vi "ADIS16470 Loop.vi"(8 "error in":errorcluster) -> ()   [LabVIEW 2025]
uses:
  <vilib>/Rock Robotics/WPI/ThirdParty/ADI/ADIS16470/Typedef/ADIS16470 Device Reference.ctl
  <vilib>/Rock Robotics/WPI/ThirdParty/ADI/ADIS16470/Typedef/ADIS16470 Hardware Configuration.ctl
  <vilib>/Rock Robotics/WPI/SPI/WPI_SPIMode.ctl
  <vilib>/Rock Robotics/SystemInterfaces/DIO/FPGA_DIOChannel.ctl
  <vilib>/Rock Robotics/SystemInterfaces/spilib/spi_bus.ctl
  <vilib>/Rock Robotics/WPI/ThirdParty/ADI/ADIS16470/Typedef/ADIS16470 Status.ctl
  <vilib>/Rock Robotics/WPI/ThirdParty/ADI/ADIS16470/Typedef/ADIS16470 Data.ctl
  <vilib>/Rock Robotics/WPI/ThirdParty/ADI/ADIS16470/Typedef/ADIS16470 Process.ctl
  <vilib>/Rock Robotics/WPI/ThirdParty/ADI/ADIS16470/Typedef/ADIS16470 Command Type.ctl
  <vilib>/Rock Robotics/SystemInterfaces/CounterEncoderSourceConvertion/FPGA_CounterEncoderSourceConvertionLVSourceType.ctl
  <vilib>/Rock Robotics/SystemInterfaces/DIO/FPGA_DIODigitalSourceChannel.ctl
  <vilib>/Rock Robotics/SystemInterfaces/AnalogTrigger/FPGA_AnalogTriggerIndex.ctl
  <vilib>/Rock Robotics/SystemInterfaces/AnalogTrigger/FPGA_AnalogTriggerOutType.ctl
  <vilib>/Rock Robotics/WPI/SPI/WPI_SPIDevRef.ctl
  <vilib>/Rock Robotics/WPI/ThirdParty/ADI/ADIS16470/Typedef/ADIS16470 Register.ctl
  <vilib>/Rock Robotics/WPI/Counter/WPI_CounterDigitalInputToDigitalSource.vi
panel:
  out "Offset Bias":i16[](array[numeric])
  in  "ADIS16470DevRef":T1={"DevStatus"={"status"=FALSE, "code"=0, "source"=""}, "Hardware Config"={"SPI Clock Rate (Hz)"=1000000.0, "IMU SPI Mode (3)"=enum."Mode 3 (Clk Idle High,Sample on Trailing)", "IMU Reset Pin"=enum."SPI Port CS2", "IMU SPI Bus"=enum."SPI On-Board, CS0", "IMU Data Ready Pin"=enum."SPI Port CS1", "Stall Config"={"Pow2BytesPerRead"=255, "StallTicks"=640, "CsToSclkTicks"=5}}, "Calibration Complete"=refnum, "Status Reference"=refnum, "Data Reference"=refnum, "Sychronous Process VI"=refnum, "Cmd FIFO"=refnum, "Source"={"DevStatus"={"status"=FALSE, "code"=0, "source"=""}, "AnalogTriggerMode?"=FALSE, "DigitalMode"={"DIO Channel"=enum."Disabled"}, "AnalogTriggerMode"={"AnalogTriggerIndex"=enum."Trig 0", "OutputType"=enum."InWindow"}}, "Data FIFO"=refnum, "Calibration Time (ms)"=5, "Data Reference"=refnum}
  in  "Main Name":string
  # "XG_BIAS_LOW"
  # "XG_BIAS_HIGH"
  # "YG_BIAS_LOW"
  # "YG_BIAS_HIGH"
  # "ZG_BIAS_LOW"
  # "ZG_BIAS_HIGH"
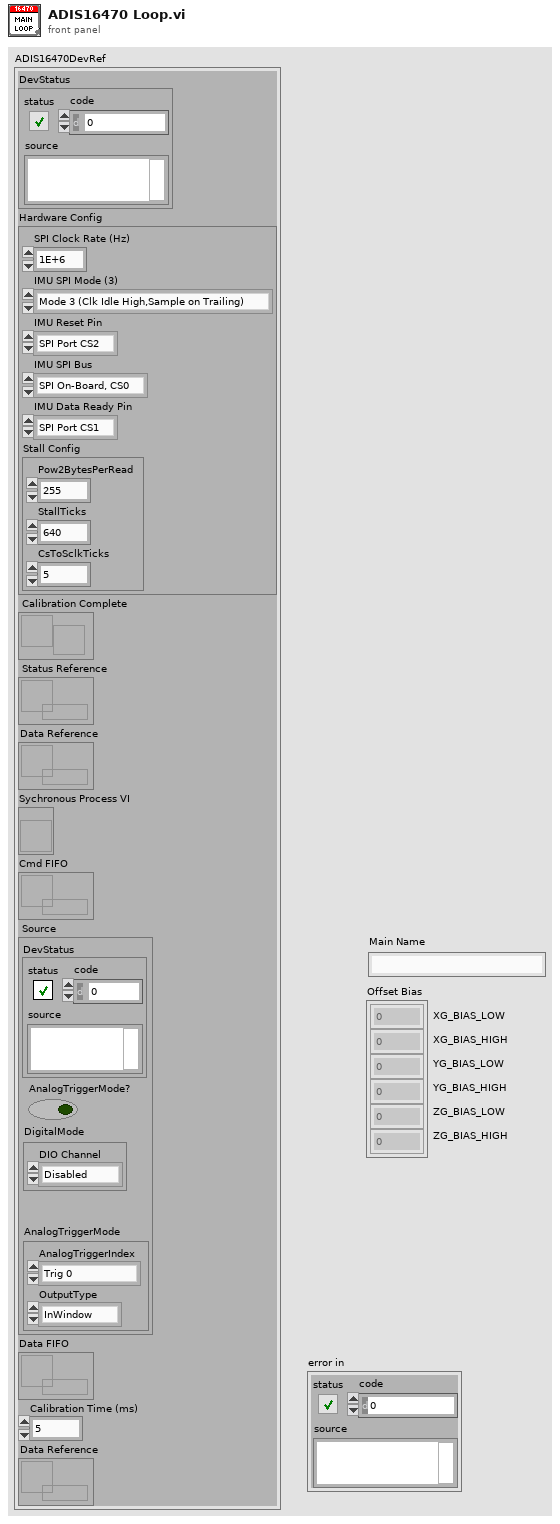
[diagram p1: front panel]
types:
  T1 = typedef "ADIS16470 Device Reference.ctl" = cluster{"DevStatus":errorcluster, "Hardware Config":T2, "Calibration Complete":refnum<notifier>, "Status Reference":refnum<data-value>, "Data Reference":refnum<data-value>, "Sychronous Process VI":T6, "Cmd FIFO":refnum<k33>, "Source":T7, "Data FIFO":refnum<k33>, "Calibration Time (ms)":u32, "Data Reference":refnum<data-value>}
  T2 = typedef "ADIS16470 Hardware Configuration.ctl" = cluster{"SPI Clock Rate (Hz)":dbl, "IMU SPI Mode (3)":T3, "IMU Reset Pin":T4, "IMU SPI Bus":T5, "IMU Data Ready Pin":T4, "Stall Config":cluster{"Pow2BytesPerRead":u8, "StallTicks":u16, "CsToSclkTicks":u8}}
  T3 = typedef "WPI_SPIMode.ctl" = enum16{"Mode 0 (Clk Idle Low,Sample on Leading)", "Mode 1 (Clk Idle Low,Sample on Trailing)", "Mode 2 (Clk Idle High,Sample on Leading)", "Mode 3 (Clk Idle High,Sample on Trailing)"}
  T4 = typedef "FPGA_DIOChannel.ctl" = enum8{"DIO 0", "DIO 1", "DIO 2", "DIO 3", "DIO 4", "DIO 5", "DIO 6", "DIO 7", "DIO 8", "DIO 9", "DIO MXP 0", "DIO MXP 1", "DIO MXP 2", "DIO MXP 3", "DIO MXP 4", "DIO MXP 5", "DIO MXP 6", "DIO MXP 7", "DIO MXP 8", "DIO MXP 9", "DIO MXP 10", "DIO MXP 11", "DIO MXP 12", "DIO MXP 13", "DIO MXP 14", "DIO MXP 15", "SPI Port CS1", "SPI Port CS2", "SPI Port CS3", "SPI Port MISO", "SPI Port MOSI", "Invalid"}
  T5 = typedef "spi_bus.ctl" = enum16{"SPI On-Board, CS0", "SPI On-Board, CS1", "SPI On-Board, CS2", "SPI On-Board, CS3", "SPI MXP", "Invalid"}
  T6 = typedef "ADIS16470 Process.ctl" = refnum<vi>
  T7 = typedef "FPGA_CounterEncoderSourceConvertionLVSourceType.ctl" = cluster{"DevStatus":errorcluster, "AnalogTriggerMode?":bool, "DigitalMode":cluster{"DIO Channel":T8}, "AnalogTriggerMode":cluster{"AnalogTriggerIndex":T9, "OutputType":T10}}
  T8 = typedef "FPGA_DIODigitalSourceChannel.ctl" = enum8{"DIO 0", "DIO 1", "DIO 2", "DIO 3", "DIO 4", "DIO 5", "DIO 6", "DIO 7", "DIO 8", "DIO 9", "DIO MXP 0", "DIO MXP 1", "DIO MXP 2", "DIO MXP 3", "DIO MXP 4", "DIO MXP 5", "DIO MXP 6", "DIO MXP 7", "DIO MXP 8", "DIO MXP 9", "DIO MXP 10", "DIO MXP 11", "DIO MXP 12", "DIO MXP 13", "DIO MXP 14", "DIO MXP 15", "SPI Port CS1", "SPI Port CS2", "SPI Port CS3", "SPI Port MISO", "SPI Port MOSI", "Disabled"}
  T9 = typedef "FPGA_AnalogTriggerIndex.ctl" = enum8{"Trig 0", "Trig 1", "Trig 2", "Trig 3", "Trig 4", "Trig 5", "Trig 6", "Trig 7", "Invalid"}
  T10 = typedef "FPGA_AnalogTriggerOutType.ctl" = enum16{"InWindow", "TriggerState", "Rising", "Falling"}
  T11 = typedef "WPI_SPIDevRef.ctl" = cluster{"DevStatus":errorcluster, "Handle":i32, "SPI Bus":T5}
  T12 = typedef "ADIS16470 Data.ctl" = cluster{"XAngle":dbl, "YAngle":dbl, "ZAngle":dbl}
  T13 = typedef "ADIS16470 Register.ctl" = u8
  T14 = cluster{"SPIDevRef":T11, "Data Counter":u16, "Reset":bool, "Digital Source":T7, "Bytes Per Sample":u32, "Data":T12, "ADIS16470DevRef":T1, "TimeStampPrev":u32, "Sensor to Robot Rotation":dbl[][], "Data Packet":T13[], "AutoSPI Active?":bool, "Delay Factor":dbl}
  T15 = typedef "ADIS16470 Status.ctl" = cluster{"Calibrated?":bool, "IMU Detected?":bool}
  T16 = typedef "ADIS16470 Command Type.ctl" = cluster{"Command":enum16{"None", "Reset", "Recalibrate"}, "Data":u32}
  T17 = typedef "WPI_DigitalOutputDevRef.ctl" = cluster{"DIO Channel":T4, "DevStatus":errorcluster}
  T18 = typedef "WPI_DigitalInputDevRef.ctl" = cluster{"DevStatus":errorcluster, "DIO Channel":T4}
  T19 = cluster{"Pow2BytesPerRead":u8, "StallTicks":u16, "CsToSclkTicks":u8}
  T20 = enum32{"Bad", "Idle", "Run top level", "Running"}
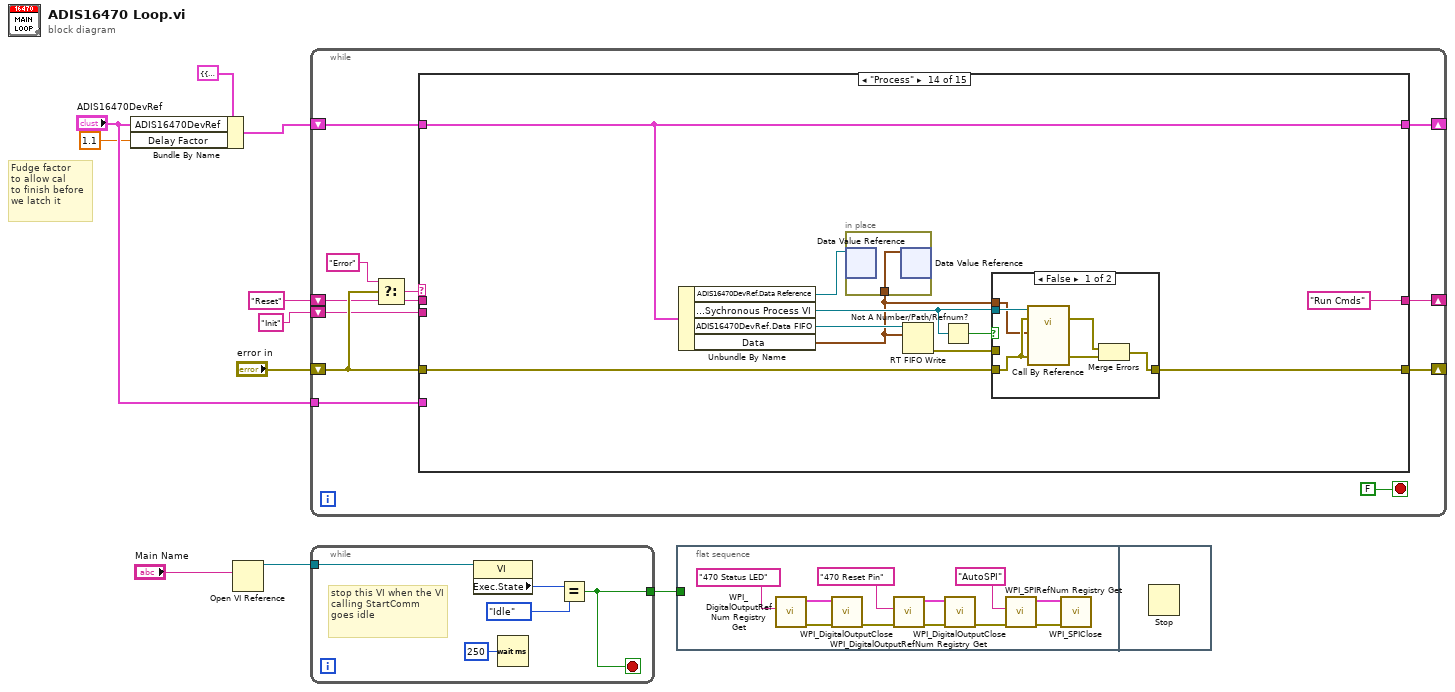
[diagram p0: block diagram]
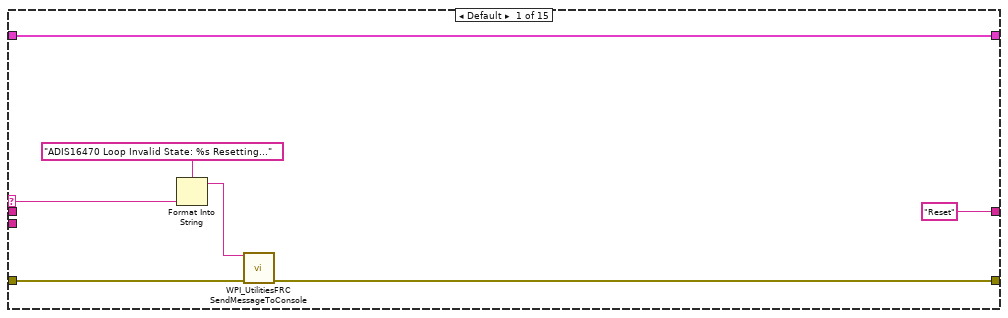
[diagram p2: hidden frame]
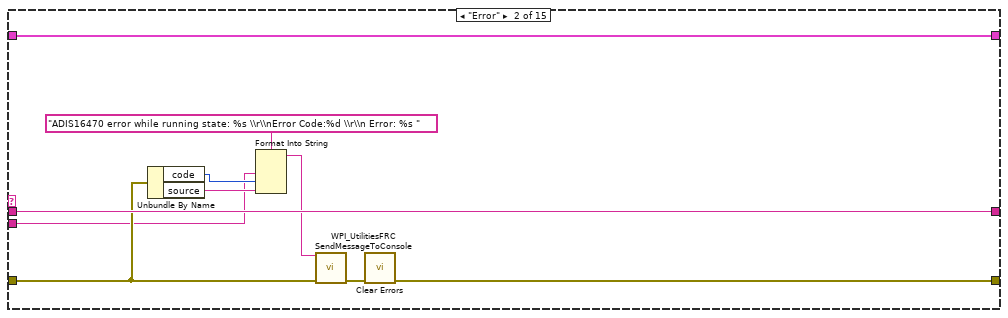
[diagram p3: hidden frame]
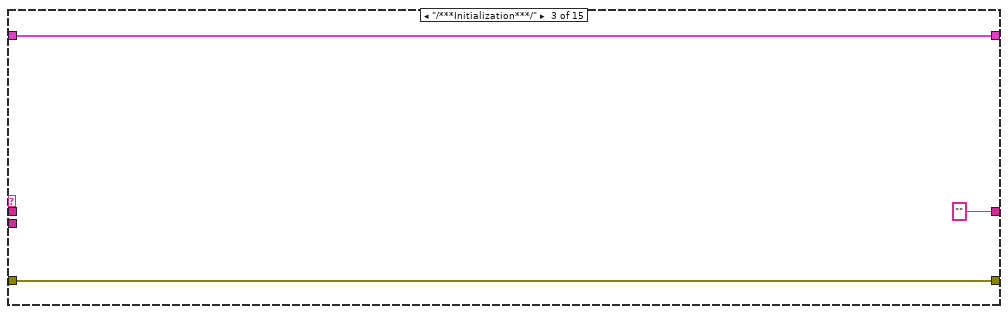
[diagram p4: hidden frame]
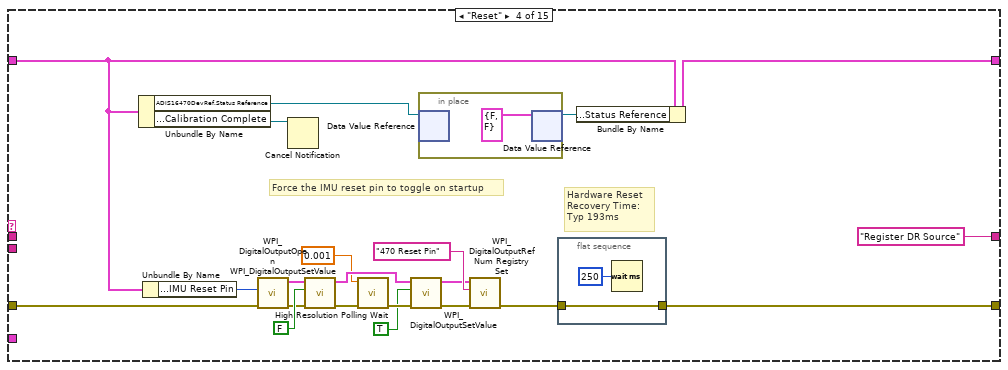
[diagram p5: hidden frame]
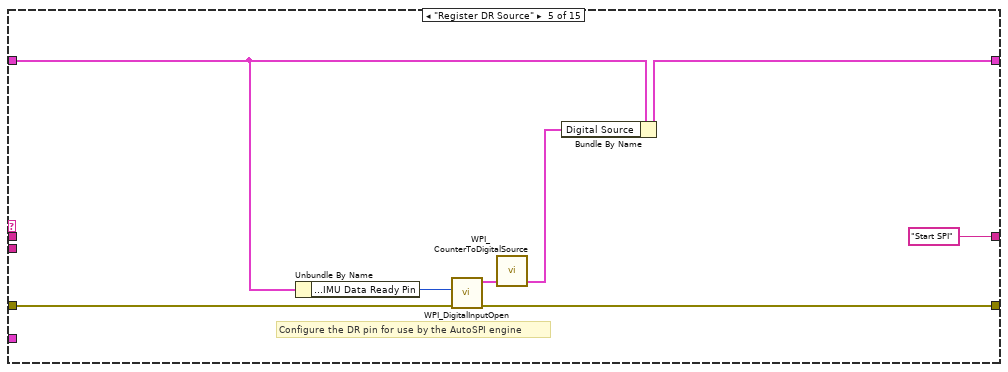
[diagram p6: hidden frame]
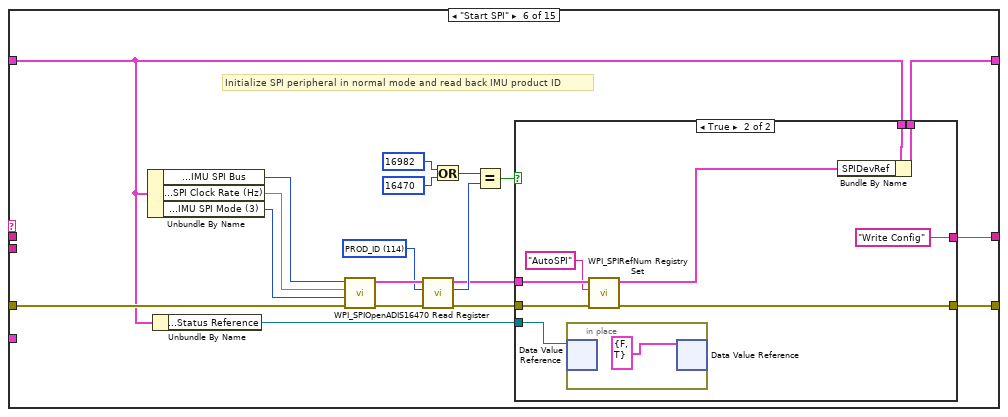
[diagram p7: hidden frame]
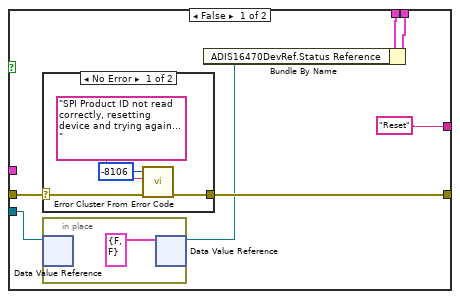
[diagram p8: hidden frame]
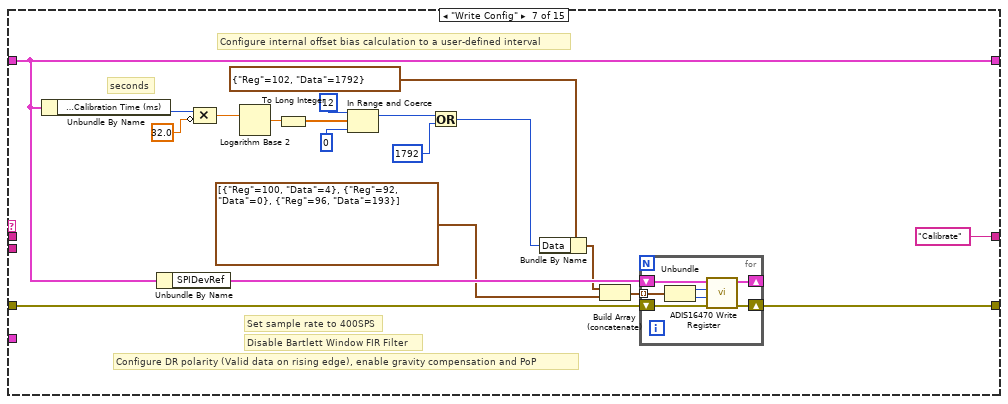
[diagram p10: hidden frame]
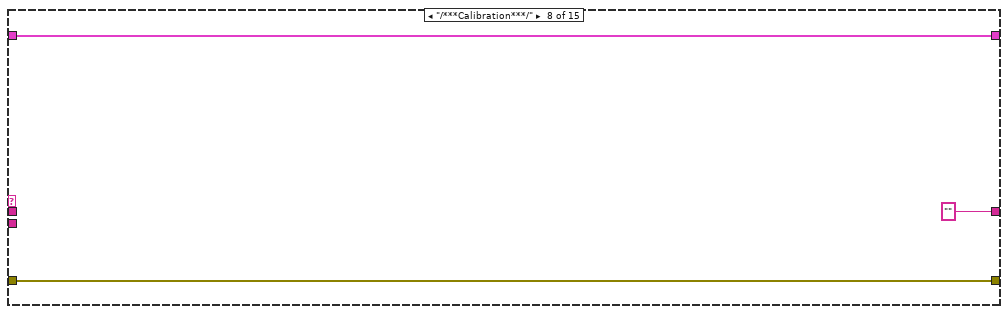
[diagram p11: hidden frame]
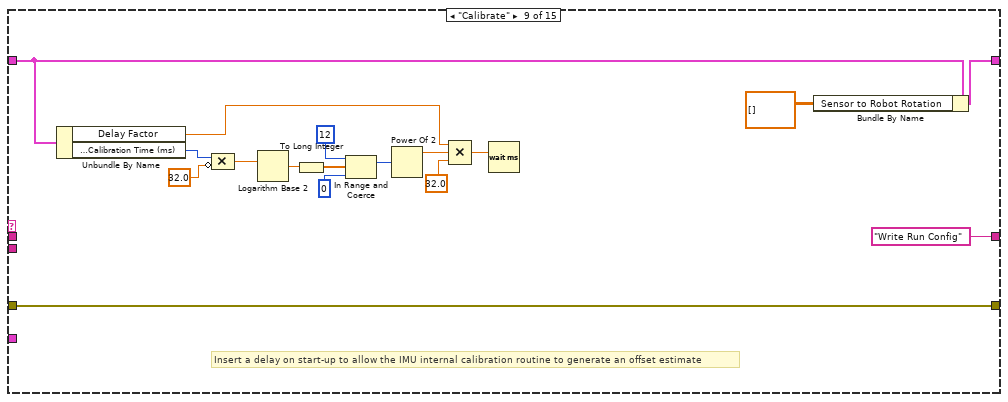
[diagram p12: hidden frame]
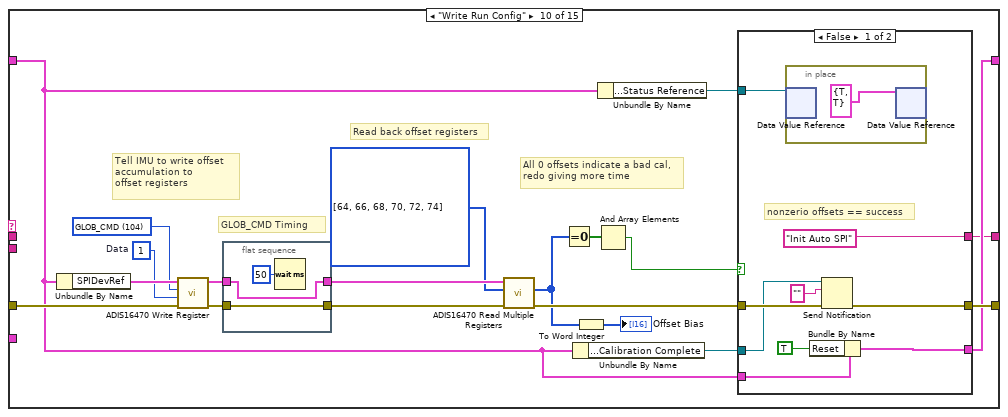
[diagram p13: hidden frame]
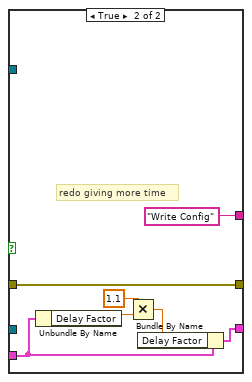
[diagram p14: hidden frame]
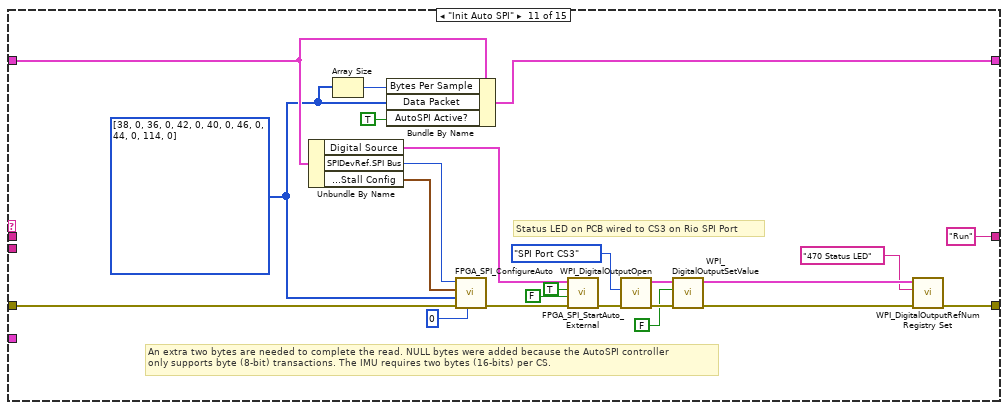
[diagram p15: hidden frame]
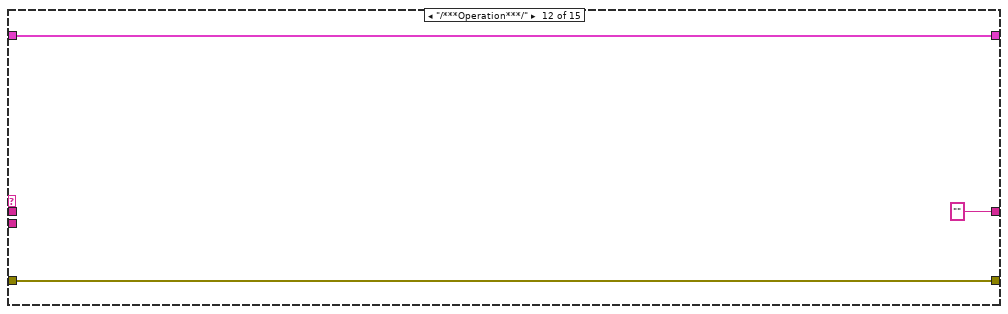
[diagram p16: hidden frame]
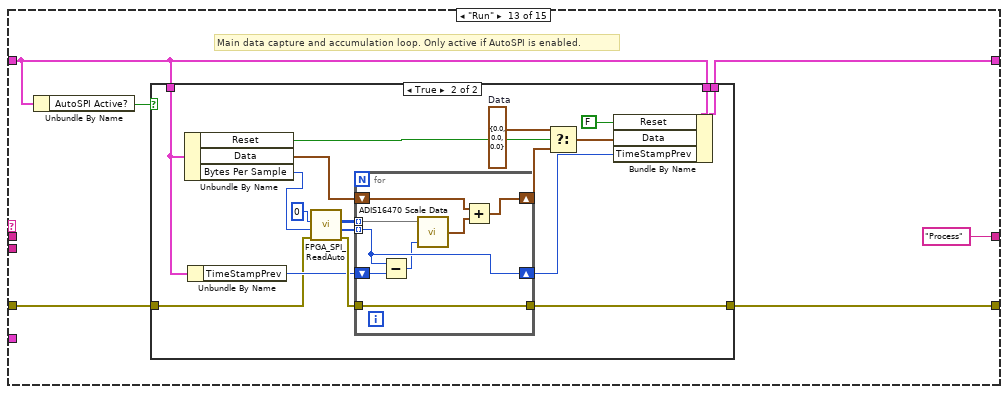
[diagram p17: hidden frame]
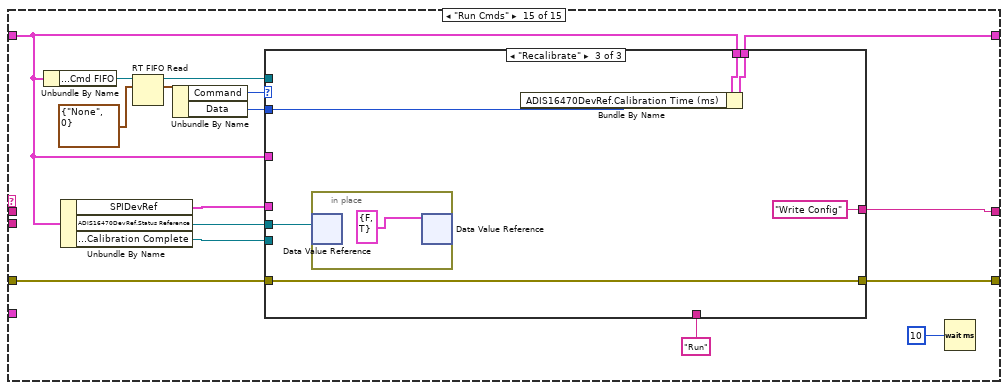
[diagram p20: hidden frame]
diagram:
  # "Fudge factor\nto allow cal\nto finish before\nwe latch it"
  n1 = Bundle By Name(cluster=T14 {"SPIDevRef"={"DevStatus"={"status"=FALSE, "code"=0, "source"=""}, "Handle"=0, "SPI Bus"=enum."SPI On-Board, CS0"}, "Data Counter"=0, "Reset"=FALSE, "Digital Source"={"DevStatus"={"status"=FALSE, "code"=0, "source"=""}, "AnalogTriggerMode?"=FALSE, "DigitalMode"={"DIO Channel"=enum."DIO 1"}, "AnalogTriggerMode"={"AnalogTriggerIndex"=enum."Trig 0", "OutputType"=enum."InWindow"}}, "Bytes Per Sample"=0, "Data"={"XAngle"=0.0, "YAngle"=0.0, "ZAngle"=0.0}, "ADIS16470DevRef"={"DevStatus"={"status"=FALSE, "code"=0, "source"=""}, "Hardware Config"={"SPI Clock Rate (Hz)"=1000000.0, "IMU SPI Mode (3)"=enum."Mode 3 (Clk Idle High,Sample on Trailing)", "IMU Reset Pin"=enum."SPI Port CS2", "IMU SPI Bus"=enum."SPI On-Board, CS0", "IMU Data Ready Pin"=enum."SPI Port CS1", "Stall Config"={"Pow2BytesPerRead"=255, "StallTicks"=640, "CsToSclkTicks"=5}}, "Calibration Complete"=refnum, "Status Reference"=refnum, "Data Reference"=refnum, "Sychronous Process VI"=refnum, "Cmd FIFO"=refnum, "Source"={"DevStatus"={"status"=FALSE, "code"=0, "source"=""}, "AnalogTriggerMode?"=FALSE, "DigitalMode"={"DIO Channel"=enum."Disabled"}, "AnalogTriggerMode"={"AnalogTriggerIndex"=enum."Trig 0", "OutputType"=enum."InWindow"}}, "Data FIFO"=refnum, "Calibration Time (ms)"=5, "Data Reference"=refnum}, "TimeStampPrev"=0, "Sensor to Robot Rotation"=[], "Data Packet"=[38, 0, 36, 0, 42, 0, 40, 0, 46, 0, 44, 0, 114, 0], "AutoSPI Active?"=TRUE, "Delay Factor"=1.1}, "ADIS16470DevRef"="ADIS16470DevRef", "Delay Factor"=1.1) -> (w6:T14)
  n2 = Open VI Reference(vi path="Main Name") -> (vi reference=w9:refnum<vi>)  [unwired: 3 in, 3 out]
  n3 = while {
    shift-right: [w17] -> _
    shift-left: "Reset" -> [w14]
    shift-right: [w19] -> _
    shift-left: w6 -> [w20]
    shift-right: [w18] -> _
    shift-left: "error in" -> [w16]
    shift-left: "Init" -> [w12]
    tunnel: "ADIS16470DevRef" -> [w11]
    stop <- FALSE stop-if-true
    n4 = Select(t="Error", s=w16, f=w14) -> (s? t:f=w15:string)
    n5 = case shown="\"Process\"" w15 {
      selector: w15 -> [w27 _ _ _ _ _ _ _ _ _ _ _ _ _ _]
      tunnel: w20 -> [w28 w38 w41 w45 w69 w75 w124 w144 w157 w164 w216 w227 w229 w270 w284]
      tunnel: [w28 w38 w41 w44 w72 w83 w124 w144 w160 w165 w215 w227 w232 w270 w291] -> w19
      tunnel: w16 -> [w26 w34 w40 w60 w71 w89 w132 w143 w159 w180 w223 w226 w231 w268 w293]
      tunnel: [w25 w35 w40 w58 w66 w82 w131 w143 w159 w171 w207 w226 w230 w267 w292] -> w18
      tunnel: ["Reset" w37 "" "Register DR Source" "Start SPI" w84 "Calibrate" "" "Write Run Config" w163 "Run" "" "Process" "Run Cmds" w281] -> w17
      tunnel: w14 -> [_ w37 _ _ _ _ _ _ _ _ _ _ _ _ _]
      tunnel: w12 -> [_ w29 _ _ _ _ _ _ _ _ _ _ _ _ _]
      tunnel: w11 -> [_ _ _ _ _ _ _ _ _ _ _ _ _ _ _]
      frame Default {
        n6 = Format Into String(format string="ADIS16470 Loop Invalid State: %s Resetting...", w27) -> (resulting string=w24:string)  [unwired: 2 in, 1 out]
        n7 = call <vilib>:"WPI_UtilitiesFRC SendMessageToConsole.vi"("Message"=w24, "error in (no error)"=w26) -> ("error out"=w25:errorcluster)  [unwired: 13 in]
      }
      frame "Error" {
        n8 = Unbundle By Name(w34) -> ("code"=w31:i32, "source"=w30:string)
        n9 = Format Into String(format string="ADIS16470 error while running state: %s \\r\\nError Code:%d \\r\\n Error: %s ", w29, w31, w30) -> (resulting string=w33:string)  [unwired: 2 in, 1 out]
        n10 = call <vilib>:"WPI_UtilitiesFRC SendMessageToConsole.vi"("Message"=w33, "error in (no error)"=w34) -> ("error out"=w36:errorcluster)  [unwired: 13 in]
        n11 = call <vilib>:"Clear Errors.vi"("error in (no error)"=w36) -> ("error out"=w35:errorcluster)  [unwired: 5 in, 1 out]
      }
      frame "/***Initialization***/" {
      }
      frame "Reset" {
        # "Hardware Reset Recovery Time: Typ 193ms"
        # "Force the IMU reset pin to toggle on startup"
        n12 = Unbundle By Name(w45) -> ("ADIS16470DevRef.Status Reference"=w43:refnum<data-value>, "ADIS16470DevRef.Calibration Complete"=w57:refnum<notifier>)
        n13 = Unbundle By Name(w45) -> ("ADIS16470DevRef.Hardware Config.IMU Reset Pin"=w61:T4)
        n14 = call <vilib>:"WPI_DigitalOutputOpen.vi"("error in (no error)"=w60, "DIO Channel"=w61) -> ("error out"=w55:errorcluster, "DigitalOutputDevRef"=w62:T17)  [unwired: 8 in]
        n15 = Cancel Notification(0:w57) -> ()  [unwired: 1 in, 3 out]
        n16 = call <vilib>:"WPI_DigitalOutputSetValue.vi"("error in (no error)"=w55, "Value"=FALSE, "DigitalOutputDevRef"=w62) -> ("error out"=w52:errorcluster, "DigitalOutputDevRef"=w50:T17)  [unwired: 7 in]
        n17 = call <vilib>:"High Resolution Polling Wait.vi"("error in (no error)"=w52, "seconds to wait"=0.001) -> ("error out"=w51:errorcluster)  [unwired: 9 in]
        n18 = call <vilib>:"WPI_DigitalOutputSetValue.vi"("error in (no error)"=w51, "Value"=TRUE, "DigitalOutputDevRef"=w50) -> ("error out"=w47:errorcluster, "DigitalOutputDevRef"=w48:T17)  [unwired: 7 in]
        n19 = in-place {
          n20 = in-place-dvr #1(w43) -> ()  [unwired: 2 out]
          n21 = in-place-dvr #1(T15 {"Calibrated?"=FALSE, "IMU Detected?"=FALSE} ("element")) -> (w42:refnum<data-value>)  [unwired: 1 out]
        }
        n22 = call <vilib>:"WPI_DigitalOutputRefNum Registry Set.vi"("error in (no error)"=w47, "refnum name"="470 Reset Pin", "DigitalOutputDevRef"=w48) -> ("error out"=w53:errorcluster)  [unwired: 7 in, 1 out]
        n23 = flat-sequence {
          tunnel: [w65] -> w58
          tunnel: w53 -> [w65]
          frame #0 {
            n24 = Wait (ms)(milliseconds to wait=u32 250) -> ()  [unwired: 1 out]
          }
        }
        n25 = Bundle By Name(cluster=w45, "ADIS16470DevRef.Status Reference"=w42) -> (w44:T14)
      }
      frame "Register DR Source" {
        # "Configure the DR pin for use by the AutoSPI engine"
        n26 = Unbundle By Name(w69) -> ("ADIS16470DevRef.Hardware Config.IMU Data Ready Pin"=w68:T4)
        n27 = call <vilib>:"WPI_DigitalInputOpen.vi"("error in (no error)"=w71, "DIO Channel"=w68) -> ("error out"=w66:errorcluster, "DigitalInputDevRef"=w70:T18)  [unwired: 8 in]
        n28 = call-poly <vilib>:"WPI_CounterToDigitalSource.vi"("DigitalInputDevRef"=w70) -> ("Digital Source"=w67:T7)  [unwired: 6 in]
        n29 = Bundle By Name(cluster=w69, "Digital Source"=w67) -> (w72:T14)
      }
      frame "Start SPI" {
        w77 = T13 114 items=["Reserved1"=0, "DIAG_STAT"=2, "X_GYRO_LOW"=4, "X_GYRO_OUT"=6, "Y_GYRO_LOW"=8, "Y_GYRO_OUT"=10, "Z_GYRO_LOW"=12, "Z_GYRO_OUT"=14, "X_ACCL_LOW"=16, "X_ACCL_OUT"=18, "Y_ACCL_LOW"=20, "Y_ACCL_OUT"=22, "Z_ACCL_LOW"=24, "Z_ACCL_OUT"=26, "TEMP_OUT"=28, "TIME_STAMP"=30, "Reseved2"=32, "DATA_CNTR"=34, "X_DELTANG_LOW"=36, "X_DELTANG_OUT"=38, "Y_DELTANG_LOW"=40, "Y_DELTANG_OUT"=42, "Z_DELTANG_LOW"=44, "Z_DELTANG_OUT"=46, "X_DELTVEL_LOW"=48, "X_DELTVEL_OUT"=50, "Y_DELTVEL_LOW"=52, "Y_DELTVEL_OUT"=54, "Z_DELTVEL_LOW"=56, "Z_DELTVEL_OUT"=58, "Reserved3"=60, "Reserved4"=62, "XG_BIAS_LOW"=64, "XG_BIAS_HIGH"=66, "YG_BIAS_LOW"=68, "YG_BIAS_OUT"=70, "ZG_BIAS_LOW"=72, "ZG_BIAS_OUT"=74, "XA_BIAS_LOW"=76, "XA_BIAS_HIGH"=78, "YA_BIAS_LOW"=80, "YA_BIAS_OUT"=82, "ZA_BIAS_LOW"=84, "ZA_BIAS_OUT"=86, "Reserved5"=88, "Reserved6"=90, "FILT_CTRL"=92, "Reserved5"=94, "MSC_CTRL"=96, "UP_SCALE"=98, "DEC_RATE"=100, "NULL_CNFG"=102, "GLOB_CMD"=104, "Reserved6"=106, "FIRM_REV"=108, "FIRM_DM"=110, "FIRM_Y"=112, "PROD_ID"=114, "SERIAL_NUM"=116, "USER_SCR1"=118, "USER_SCR2"=120, "USER_SCR3"=122, "FLSHCNT_LOW"=124, "FLSHCNT_HIGH"=126] ("ADIS16448 Register")
        # "Initialize SPI peripheral in normal mode and read back IMU product ID"
        n30 = Unbundle By Name(w75) -> ("ADIS16470DevRef.Hardware Config.IMU SPI Bus"=w85:T5, "ADIS16470DevRef.Hardware Config.SPI Clock Rate (Hz)"=w86:dbl, "ADIS16470DevRef.Hardware Config.IMU SPI Mode (3)"=w87:T3)
        n31 = Unbundle By Name(w75) -> ("ADIS16470DevRef.Status Reference"=w74:refnum<data-value>)
        n32 = call <vilib>:"WPI_SPIOpen.vi"("error in"=w89, "Mode (3)"=w87, "Clock Rate (Hz)"=w86, "SPI Bus"=w85) -> ("error out"=w79:errorcluster, "SPIDevRef"=w78:T11)  [unwired: 6 in]
        n33 = call <vilib>:"ADIS16470 Read Register.vi"("error in (no error)"=w79, "ADIS16470 Register"=w77, "SPIDevRef in"=w78) -> ("error out"=w80:errorcluster, "Register Value"=w81:u16, "SPIDevRef out"=w76:T11)  [unwired: 6 in]
        n34 = Or(x=u16 16982 ("y"), y=u16 16470) -> (x .or. y?=w90:u16)
        n35 = Equal?(x=w90, y=w81) -> (x = y?=w88:bool)
        n36 = case shown="True" w88 {
          tunnel: ["Reset" "Write Config"] -> w84
          tunnel: w75 -> [w95 w113]
          tunnel: [w94 w112] -> w83
          tunnel: [w98 w108] -> w82
          tunnel: w80 -> [w97 w111]
          tunnel: w76 -> [_ w110]
          tunnel: w74 -> [w96 w106]
          frame False {
            n37 = case shown="No Error" w97 {
              selector: w97 -> [w103 w105]
              tunnel: [w104 w105] -> w98
              frame No Error {
                n38 = call <vilib>:"Error Cluster From Error Code.vi"("error in (no error)"=w103, "error message (\"\")"="SPI Product ID not read correctly, resetting device and trying again..." ("error message (\"\")"), "error code (0)"=-8106) -> ("error out"=w104:errorcluster)  [unwired: 6 in]
              }
              frame Error {
              }
            }
            n39 = in-place {
              n40 = in-place-dvr #2(w96) -> ()  [unwired: 2 out]
              n41 = in-place-dvr #2(T15 {"Calibrated?"=FALSE, "IMU Detected?"=FALSE} ("element")) -> (w93:refnum<data-value>)  [unwired: 1 out]
            }
            n42 = Bundle By Name(cluster=w95, "ADIS16470DevRef.Status Reference"=w93) -> (w94:T14)
          }
          frame True {
            n43 = in-place {
              n44 = in-place-dvr #3(w106) -> ()  [unwired: 2 out]
              n45 = in-place-dvr #3(T15 {"Calibrated?"=FALSE, "IMU Detected?"=TRUE} ("element")) -> ()  [unwired: 2 out]
            }
            n46 = call <vilib>:"WPI_SPIRefNum Registry Set.vi"("error in (no error)"=w111, "refnum name"="AutoSPI", "SPIDevRef"=w110) -> ("error out"=w108:errorcluster, "SPIDevRef"=w109:T11)  [unwired: 7 in]
            n47 = Bundle By Name(cluster=w113, "SPIDevRef"=w109) -> (w112:T14)
          }
        }
      }
      frame "Write Config" {
        # "seconds"
        # "Set sample rate to 400SPS"
        # "Configure internal offset bias calculation to a user-defined interval"
        # "Configure DR polarity (Valid data on rising edge), enable gravity compensation and PoP"
        # "Disable Bartlett Window FIR Filter"
        n48 = Unbundle By Name(w124) -> ("ADIS16470DevRef.Calibration Time (ms)"=w119:u32)
        n49 = Unbundle By Name(w124) -> ("SPIDevRef"=w133:T11)
        n50 = Compound Arithmetic op=MULTIPLY(w119, invert 32.0 ("x")) -> (w117:dbl)
        n51 = Logarithm Base 2(1:w117) -> (0:w123:dbl)
        n52 = To Long Integer(number=w123) -> (32bit integer=w120:i32)
        n53 = In Range and Coerce(upper limit=12 ("x"), x=w120, lower limit=0 ("x")) -> (coerced(x)=w116:i32)  [unwired: 1 out]
        n54 = Or(x=w116, y=1792 ("Data")) -> (x .or. y?=w125:i32)
        n55 = Bundle By Name(cluster=cluster{"Reg":T13, "Data":i32} {"Reg"=102, "Data"=1792}, "Data"=w125) -> (w127:cluster{"Reg":T13, "Data":i32})
        n56 = Build Array (concatenate)(w127, cluster{"Reg":T13, "Data":u16}[] [{"Reg"=100, "Data"=4}, {"Reg"=92, "Data"=0}, {"Reg"=96, "Data"=193}]) -> (w128:cluster{"Reg":T13, "Data":i32}[])
        n57 = for {
          tunnel: w128 -> [w141] mode=indexing
          shift-right: [w137] -> w131
          shift-left: w132 -> [w136]
          shift-right: [w135] -> _
          shift-left: w133 -> [w138]
          n58 = Unbundle(w141) -> ("Reg"=w140:T13, "Data"=w139:i32)
          n59 = call <vilib>:"ADIS16470 Write Register.vi"("error in (no error)"=w136, "Data"=w139, "Register"=w140, "SPIDevRef in"=w138) -> ("error out"=w137:errorcluster, "SPIDevRef out"=w135:T11)  [unwired: 6 in]
        }
      }
      frame "/***Calibration***/" {
      }
      frame "Calibrate" {
        # "Insert a delay on start-up to allow the IMU internal calibration routine to generate an offset estimate"
        n60 = Unbundle By Name(w157) -> ("Delay Factor"=w145:dbl, "ADIS16470DevRef.Calibration Time (ms)"=w151:u32)
        n61 = Compound Arithmetic op=MULTIPLY(w151, invert 32.0 ("x")) -> (w152:dbl)
        n62 = Logarithm Base 2(1:w152) -> (0:w156:dbl)
        n63 = To Long Integer(number=w156) -> (32bit integer=w154:i32)
        n64 = In Range and Coerce(upper limit=12 ("x"), x=w154, lower limit=0 ("x")) -> (coerced(x)=w149:i32)  [unwired: 1 out]
        n65 = Power Of 2(x=w149) -> (2^x=w148:dbl)
        n66 = Compound Arithmetic op=MULTIPLY(w145, w148, 32.0 ("x")) -> (w146:dbl)
        n67 = Wait (ms)(milliseconds to wait=w146) -> ()  [unwired: 1 out]
        n68 = Bundle By Name(cluster=w157, "Sensor to Robot Rotation"=dbl[][] []) -> (w160:T14)
      }
      frame "Write Run Config" {
        w170 = T13 104 items=["Reserved1"=0, "DIAG_STAT"=2, "X_GYRO_LOW"=4, "X_GYRO_OUT"=6, "Y_GYRO_LOW"=8, "Y_GYRO_OUT"=10, "Z_GYRO_LOW"=12, "Z_GYRO_OUT"=14, "X_ACCL_LOW"=16, "X_ACCL_OUT"=18, "Y_ACCL_LOW"=20, "Y_ACCL_OUT"=22, "Z_ACCL_LOW"=24, "Z_ACCL_OUT"=26, "TEMP_OUT"=28, "TIME_STAMP"=30, "Reseved2"=32, "DATA_CNTR"=34, "X_DELTANG_LOW"=36, "X_DELTANG_OUT"=38, "Y_DELTANG_LOW"=40, "Y_DELTANG_OUT"=42, "Z_DELTANG_LOW"=44, "Z_DELTANG_OUT"=46, "X_DELTVEL_LOW"=48, "X_DELTVEL_OUT"=50, "Y_DELTVEL_LOW"=52, "Y_DELTVEL_OUT"=54, "Z_DELTVEL_LOW"=56, "Z_DELTVEL_OUT"=58, "Reserved3"=60, "Reserved4"=62, "XG_BIAS_LOW"=64, "XG_BIAS_HIGH"=66, "YG_BIAS_LOW"=68, "YG_BIAS_OUT"=70, "ZG_BIAS_LOW"=72, "ZG_BIAS_OUT"=74, "XA_BIAS_LOW"=76, "XA_BIAS_HIGH"=78, "YA_BIAS_LOW"=80, "YA_BIAS_OUT"=82, "ZA_BIAS_LOW"=84, "ZA_BIAS_OUT"=86, "Reserved5"=88, "Reserved6"=90, "FILT_CTRL"=92, "Reserved5"=94, "MSC_CTRL"=96, "UP_SCALE"=98, "DEC_RATE"=100, "NULL_CNFG"=102, "GLOB_CMD"=104, "Reserved6"=106, "FIRM_REV"=108, "FIRM_DM"=110, "FIRM_Y"=112, "PROD_ID"=114, "SERIAL_NUM"=116, "USER_SCR1"=118, "USER_SCR2"=120, "USER_SCR3"=122, "FLSHCNT_LOW"=124, "FLSHCNT_HIGH"=126] ("Register")
        w179 = u16 1  # Data
        w175 = T13[] [64, 66, 68, 70, 72, 74] items=["Reserved1"=0, "DIAG_STAT"=2, "X_GYRO_LOW"=4, "X_GYRO_OUT"=6, "Y_GYRO_LOW"=8, "Y_GYRO_OUT"=10, "Z_GYRO_LOW"=12, "Z_GYRO_OUT"=14, "X_ACCL_LOW"=16, "X_ACCL_OUT"=18, "Y_ACCL_LOW"=20, "Y_ACCL_OUT"=22, "Z_ACCL_LOW"=24, "Z_ACCL_OUT"=26, "TEMP_OUT"=28, "TIME_STAMP"=30, "Reseved2"=32, "DATA_CNTR"=34, "X_DELTANG_LOW"=36, "X_DELTANG_OUT"=38, "Y_DELTANG_LOW"=40, "Y_DELTANG_OUT"=42, "Z_DELTANG_LOW"=44, "Z_DELTANG_OUT"=46, "X_DELTVEL_LOW"=48, "X_DELTVEL_OUT"=50, "Y_DELTVEL_LOW"=52, "Y_DELTVEL_OUT"=54, "Z_DELTVEL_LOW"=56, "Z_DELTVEL_OUT"=58, "Reserved3"=60, "Reserved4"=62, "XG_BIAS_LOW"=64, "XG_BIAS_HIGH"=66, "YG_BIAS_LOW"=68, "YG_BIAS_HIGH"=70, "ZG_BIAS_LOW"=72, "ZG_BIAS_HIGH"=74, "XA_BIAS_LOW"=76, "XA_BIAS_HIGH"=78, "YA_BIAS_LOW"=80, "YA_BIAS_HIGH"=82, "ZA_BIAS_LOW"=84, "ZA_BIAS_HIGH"=86, "Reserved5"=88, "Reserved6"=90, "FILT_CTRL"=92, "Reserved5"=94, "MSC_CTRL"=96, "UP_SCALE"=98, "DEC_RATE"=100, "NULL_CNFG"=102, "GLOB_CMD"=104, "Reserved6"=106, "FIRM_REV"=108, "FIRM_DM"=110, "FIRM_Y"=112, "PROD_ID"=114, "SERIAL_NUM"=116, "USER_SCR1"=118, "USER_SCR2"=120, "USER_SCR3"=122, "FLSHCNT_LOW"=124, "FLSHCNT_HIGH"=126] ("Registers")
        # "All 0 offsets indicate a bad cal,\nredo giving more time"
        # "Tell IMU to write offset \naccumulation to \noffset registers"
        # "GLOB_CMD Timing"
        # "Read back offset registers"
        n69 = Unbundle By Name(w164) -> ("SPIDevRef"=w181:T11)
        n70 = call <vilib>:"ADIS16470 Write Register.vi"("error in (no error)"=w180, "Data"=w179, "Register"=w170, "SPIDevRef in"=w181) -> ("error out"=w178:errorcluster, "SPIDevRef out"=w177:T11)  [unwired: 6 in]
        n71 = flat-sequence {
          tunnel: w178 -> [w201]
          tunnel: [w201] -> w169
          tunnel: w177 -> [w199]
          tunnel: [w199] -> w176
          frame #0 {
            n72 = Wait (ms)(milliseconds to wait=u32 50) -> ()  [unwired: 1 out]
          }
        }
        n73 = call <vilib>:"ADIS16470 Read Multiple Registers.vi"("error in (no error)"=w169, "Registers"=w175, "SPIDevRefIn"=w176) -> ("error out"=w173:errorcluster, "Values"=w168:u16[])  [unwired: 6 in, 1 out]
        n74 = Equal To 0?(x=w168) -> (x = 0?=w167:bool[])
        n75 = Unbundle By Name(w164) -> ("ADIS16470DevRef.Calibration Complete"=w172:refnum<notifier>)
        n76 = To Word Integer(number=w168) -> (16bit integer=→"Offset Bias":i16[])
        n77 = Unbundle By Name(w164) -> ("ADIS16470DevRef.Status Reference"=w162:refnum<data-value>)
        n78 = And Array Elements(Boolean array=w167) -> (logical AND=w166:bool)
        n79 = case shown="False" w166 {
          tunnel: w173 -> [w190 w198]
          tunnel: w172 -> [w189 _]
          tunnel: [w188 w198] -> w171
          tunnel: w164 -> [w185 w196]
          tunnel: [w184 w197] -> w165
          tunnel: ["Init Auto SPI" "Write Config"] -> w163
          tunnel: w162 -> [w182 _]
          frame False {
            # "nonzerio offsets == success"
            n80 = in-place {
              n81 = in-place-dvr #4(w182) -> ()  [unwired: 2 out]
              n82 = in-place-dvr #4(T15 {"Calibrated?"=TRUE, "IMU Detected?"=TRUE} ("element")) -> ()  [unwired: 2 out]
            }
            n83 = Bundle By Name(cluster=w185, "Reset"=TRUE ("First Run")) -> (w184:T14)
            n84 = Send Notification(notification="", notifier=w189, error in (no error)=w190) -> (error out=w188:errorcluster)  [unwired: 1 out]
          }
          frame True {
            # "redo giving more time"
            n85 = Unbundle By Name(w196) -> ("Delay Factor"=w195:dbl)
            n86 = Multiply(x=1.1, y=w195) -> (x*y=w193:dbl)
            n87 = Bundle By Name(cluster=w196, "Delay Factor"=w193) -> (w197:T14)
          }
        }
      }
      frame "Init Auto SPI" {
        w202 = T13[] [38, 0, 36, 0, 42, 0, 40, 0, 46, 0, 44, 0, 114, 0] items=["NULL"=0, "DIAG_STAT"=2, "X_GYRO_LOW"=4, "X_GYRO_OUT"=6, "Y_GYRO_LOW"=8, "Y_GYRO_OUT"=10, "Z_GYRO_LOW"=12, "Z_GYRO_OUT"=14, "X_ACCL_LOW"=16, "X_ACCL_OUT"=18, "Y_ACCL_LOW"=20, "Y_ACCL_OUT"=22, "Z_ACCL_LOW"=24, "Z_ACCL_OUT"=26, "TEMP_OUT"=28, "TIME_STAMP"=30, "Reseved2"=32, "DATA_CNTR"=34, "X_DELTANG_LOW"=36, "X_DELTANG_OUT"=38, "Y_DELTANG_LOW"=40, "Y_DELTANG_OUT"=42, "Z_DELTANG_LOW"=44, "Z_DELTANG_OUT"=46, "X_DELTVEL_LOW"=48, "X_DELTVEL_OUT"=50, "Y_DELTVEL_LOW"=52, "Y_DELTVEL_OUT"=54, "Z_DELTVEL_LOW"=56, "Z_DELTVEL_OUT"=58, "Reserved3"=60, "Reserved4"=62, "XG_BIAS_LOW"=64, "XG_BIAS_HIGH"=66, "YG_BIAS_LOW"=68, "YG_BIAS_HIGH"=70, "ZG_BIAS_LOW"=72, "ZG_BIAS_HIGH"=74, "XA_BIAS_LOW"=76, "XA_BIAS_HIGH"=78, "YA_BIAS_LOW"=80, "YA_BIAS_HIGH"=82, "ZA_BIAS_LOW"=84, "ZA_BIAS_HIGH"=86, "Reserved5"=88, "Reserved6"=90, "FILT_CTRL"=92, "Reserved5"=94, "MSC_CTRL"=96, "UP_SCALE"=98, "DEC_RATE"=100, "NULL_CNFG"=102, "GLOB_CMD"=104, "Reserved6"=106, "FIRM_REV"=108, "FIRM_DM"=110, "FIRM_Y"=112, "PROD_ID"=114, "SERIAL_NUM"=116, "USER_SCR1"=118, "USER_SCR2"=120, "USER_SCR3"=122, "FLSHCNT_LOW"=124, "FLSHCNT_HIGH"=126] ("Registers")
        # "Status LED on PCB wired to CS3 on Rio SPI Port"
        # "An extra two bytes are needed to complete the read. NULL bytes were added because the AutoSPI controller \nonly supports byte (8-bit) transactions. The IMU requires two bytes (16-bits) per CS."
        n88 = Unbundle By Name(w216) -> ("Digital Source"=w204:T7, "SPIDevRef.SPI Bus"=w203:T5, "ADIS16470DevRef.Hardware Config.Stall Config"=w206:T19)
        n89 = Array Size(array=w202) -> (size(s)=w214:i32)
        n90 = Bundle By Name(cluster=w216, "Bytes Per Sample"=w214, "Data Packet"=w202, "AutoSPI Active?"=TRUE) -> (w215:T14)
        n91 = call <vilib>:"FPGA_SPI_ConfigureAuto.vi"("SPI Auto Zero Byte Count"=u8 0, "error in"=w223, "SPI Auto TX Byte Array"=w202, "Stall Config"=w206, "SPI Bus"=w203) -> ("error out"=w221:errorcluster)  [unwired: 6 in]
        n92 = call <vilib>:"FPGA_SPI_StartAuto_External.vi"("error in (no error)"=w221, "Falling Edge"=FALSE, "Rising Edge"=TRUE, "Source"=w204) -> ("error out"=w217:errorcluster)  [unwired: 7 in]
        n93 = call <vilib>:"WPI_DigitalOutputOpen.vi"("error in (no error)"=w217, "DIO Channel"=FPGA_DIOChannel."SPI Port CS3") -> ("error out"=w213:errorcluster, "DigitalOutputDevRef"=w212:T17)  [unwired: 8 in]
        n94 = call <vilib>:"WPI_DigitalOutputSetValue.vi"("error in (no error)"=w213, "Value"=FALSE, "DigitalOutputDevRef"=w212) -> ("error out"=w210:errorcluster, "DigitalOutputDevRef"=w209:T17)  [unwired: 7 in]
        n95 = call <vilib>:"WPI_DigitalOutputRefNum Registry Set.vi"("error in (no error)"=w210, "refnum name"="470 Status LED", "DigitalOutputDevRef"=w209) -> ("error out"=w207:errorcluster)  [unwired: 7 in, 1 out]
      }
      frame "/***Operation***/" {
      }
      frame "Run" {
        # "Main data capture and accumulation loop. Only active if AutoSPI is enabled."
        n96 = Unbundle By Name(w229) -> ("AutoSPI Active?"=w228:bool)
        n97 = case shown="True" w228 {
          tunnel: [w235 w253] -> w232
          tunnel: w231 -> [w234 w238]
          tunnel: [w234 w243] -> w230
          tunnel: w229 -> [w235 w242]
          tunnel: w229 -> [_ w239]
          frame False {
          }
          frame True {
            w237 = T12 {"XAngle"=0.0, "YAngle"=0.0, "ZAngle"=0.0}  # Data
            n98 = Unbundle By Name(w239) -> ("Reset"=w251:bool, "Data"=w246:T12, "Bytes Per Sample"=w250:u32)
            n99 = Unbundle By Name(w239) -> ("TimeStampPrev"=w241:u32)
            n100 = call <vilib>:"FPGA_SPI_ReadAuto.vi"("error in (no error)"=w238, "Bytes per Sample"=w250, "Samples to Read"=u32 0) -> ("error out"=w244:errorcluster, "Timestamps"=w247:u32[], "Data"=w248:u8[][])  [unwired: 6 in]
            n101 = for {
              tunnel: w248 -> [w257] mode=indexing
              tunnel: w247 -> [w259] mode=indexing
              shift-right: [w256] -> w245
              shift-left: w246 -> [w261]
              tunnel: w244 -> [w258]
              tunnel: [w258] -> w243
              shift-right: [w259] -> w240
              shift-left: w241 -> [w260]
              n102 = Subtract(x=w259, y=w260) -> (x-y=w254:u32)
              n103 = call <vilib>:"ADIS16470 Scale Data.vi"("TimeStamp"=w254, "Data In"=w257) -> ("Data"=w255:T12)  [unwired: 3 in]
              n104 = Add(x=w261, y=w255) -> (x+y=w256:T12)
            }
            n105 = Select(t=w237, s=w251, f=w245) -> (s? t:f=w236:T12)
            n106 = Bundle By Name(cluster=w242, "Reset"=FALSE ("First Run"), "Data"=w236, "TimeStampPrev"=w240) -> (w253:T14)
          }
        }
      }
      frame "Process" {
        n107 = Unbundle By Name(w270) -> ("ADIS16470DevRef.Data Reference"=w264:refnum<data-value>, "ADIS16470DevRef.Sychronous Process VI"=w265:T6, "ADIS16470DevRef.Data FIFO"=w269:refnum<k33>, "Data"=w262:T12)
        n108 = in-place {
          in-place-border: w262 -> [w272]
          n109 = in-place-dvr #5(w264) -> ()  [unwired: 2 out]
          n110 = in-place-dvr #5(w272) -> ()  [unwired: 2 out]
        }
        n111 = RT FIFO Write(0:w269, 1:w262) -> (11:w263:errorcluster)  [unwired: 3 in, 3 out]
        n112 = Not A Number/Path/Refnum?(number/path/refnum=w265) -> (NaN/Path/Refnum?=w266:bool)
        n113 = case shown="False" w266 {
          tunnel: w268 -> [w274 w279]
          tunnel: [w278 w279] -> w267
          tunnel: w265 -> [w277 _]
          tunnel: w263 -> [_ _]
          tunnel: w262 -> [w273 _]
          frame False {
            n114 = call-by-ref "?"(reference=w277, error in=w274, 8:"error in (no error)"=w274, "element"=w273) -> (error out=w275:errorcluster, 0:"error out"=w276:errorcluster)  [unwired: 9 in, 1 out]
            n115 = Merge Errors(w275, w276) -> (w278:errorcluster)
          }
          frame True {
          }
        }
      }
      frame "Run Cmds" {
        n116 = Unbundle By Name(w284) -> ("ADIS16470DevRef.Cmd FIFO"=w294:refnum<k33>)
        n117 = Unbundle By Name(w284) -> ("SPIDevRef"=w283:T11, "ADIS16470DevRef.Status Reference"=w289:refnum<data-value>, "ADIS16470DevRef.Calibration Complete"=w290:refnum<notifier>)
        n118 = RT FIFO Read(0:w294, 1:T16 {"Command"=enum."None", "Data"=0} ("element")) -> (8:w288:refnum<k33>, 9:w287:T16)  [unwired: 2 in, 3 out]
        n119 = Unbundle By Name(w287) -> ("Command"=w286:enum16{"None", "Reset", "Recalibrate"}, "Data"=w285:u32)
        n120 = case shown="\"Recalibrate\"" w286 {
          tunnel: w284 -> [w297 w303 w306]
          tunnel: w293 -> [w298 w302 w308]
          tunnel: [w298 w302 w308] -> w292
          tunnel: [w297 w301 w307] -> w291
          tunnel: w290 -> [_ _ _]
          tunnel: w289 -> [_ _ w304]
          tunnel: w288 -> [_ _ _]
          tunnel: w285 -> [_ _ w305]
          tunnel: w284 -> [_ _ _]
          tunnel: w283 -> [_ _ _]
          tunnel: [w296 "Run" "Write Config"] -> w281
          tunnel: "Run" -> [w296 _ _]
          frame "None", Default {
          }
          frame "Reset" {
            n121 = Bundle By Name(cluster=w303, "Reset"=TRUE ("First Run")) -> (w301:T14)
          }
          frame "Recalibrate" {
            n122 = in-place {
              n123 = in-place-dvr #6(w304) -> ()  [unwired: 2 out]
              n124 = in-place-dvr #6(T15 {"Calibrated?"=FALSE, "IMU Detected?"=TRUE} ("element")) -> ()  [unwired: 2 out]
            }
            n125 = Bundle By Name(cluster=w306, "ADIS16470DevRef.Calibration Time (ms)"=w305) -> (w307:T14)
          }
        }
        n126 = Wait (ms)(milliseconds to wait=u32 10) -> ()  [unwired: 1 out]
      }
    }
  }
  n127 = while {
    tunnel: w9 -> [w312]
    tunnel: [w311] -> w3
    stop <- w311 stop-if-true
    # "stop this VI when the VI calling StartComm goes idle"
    n128 = property class="VI"(reference=w312) -> ("Exec.State"=w314:T20)  [unwired: 1 in, 2 out]
    n129 = Wait (ms)(milliseconds to wait=u32 250) -> ()  [unwired: 1 out]
    n130 = Equal?(x=w314, y=T20."Idle" ("Execution:State")) -> (x = y?=w311:bool)
  }
  n131 = flat-sequence {
    tunnel: w3 -> [_]
    frame #0 {
      n132 = call <vilib>:"WPI_DigitalOutputRefNum Registry Get.vi"("refnum name"="470 Status LED") -> ("error out"=w325:errorcluster, "DigitalOutputDevRef"=w324:T17)  [unwired: 9 in]
      n133 = call <vilib>:"WPI_DigitalOutputClose.vi"("error in (no error)"=w325, "DigitalOutputDevRef"=w324) -> ("error out"=w323:errorcluster)  [unwired: 9 in]
      n134 = call <vilib>:"WPI_DigitalOutputRefNum Registry Get.vi"("error in (no error)"=w323, "refnum name"="470 Reset Pin") -> ("error out"=w321:errorcluster, "DigitalOutputDevRef"=w320:T17)  [unwired: 8 in]
      n135 = call <vilib>:"WPI_DigitalOutputClose.vi"("error in (no error)"=w321, "DigitalOutputDevRef"=w320) -> ("error out"=w319:errorcluster)  [unwired: 9 in]
      n136 = call <vilib>:"WPI_SPIRefNum Registry Get.vi"("error in (no error)"=w319, "refnum name"="AutoSPI") -> ("error out"=w317:errorcluster, "SPIDevRef"=w316:T11)  [unwired: 8 in]
      n137 = call <vilib>:"WPI_SPIClose.vi"("error in (no error)"=w317, "SPIDevRef"=w316) -> ()  [unwired: 9 in, 1 out]
    }
    frame #1 {
      n138 = Stop() -> ()  [unwired: 1 in]
    }
  }
